vi "MM6.PG_Stop.vi"(0 "i ref in":refnum<vi>, 5 "error in (no error)":errorcluster) -> (14 "i ref out":refnum<vi>, 19 "error out":errorcluster)   [LabVIEW 2014, in "MM6.lvlib"]
doc: "Stops the hardware used for timing."
uses:
  MM6.lvlib
  CSCore/CSSystem/CoreLib/CoreLib.int 2 byte array.vi
  CSCore/BaseProcess/BaseProcess.lvlib
  CSCore/CSSystem/CoreLib/CoreLib.lvlib
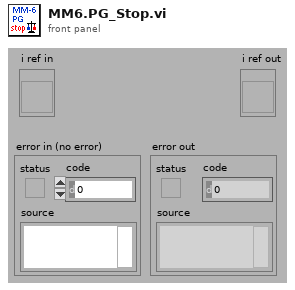
[diagram p1: front panel]
types:
  T1 = typedef "PPG_ABC.lvlib/PPG_ABC.PG_dataType.ctl" = cluster{"PGDevice":string, "rawPatternData":cluster{"triggerCondition":i32, "timeTable":dbl[], "channelTable":string[]}[]}
  T2 = typedef "CoreDefs.rawDataType.ctl" = i8[]
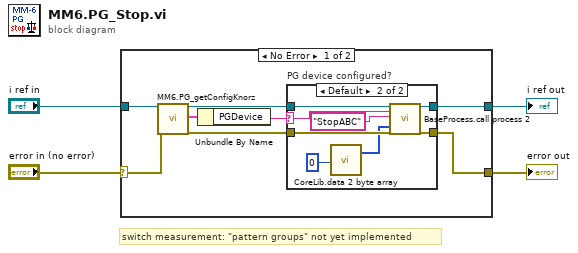
[diagram p0: block diagram]
diagram:
  # "switch measurement: \"pattern groups\" not yet implemented"
  n1 = case shown="No Error" "error in (no error)" {
    selector: "error in (no error)" -> [w11 w23]
    tunnel: "i ref in" -> [w12 w24]
    tunnel: [w7 w24] -> w3
    tunnel: [w6 w23] -> w2
    frame No Error {
      n2 = call "MM6.PG_getConfigKnorz.vi"("i ref in"=w12, "error in (no error)"=w11) -> ("i ref out"=w10:refnum<vi>, "PGData"=w8:T1, "error out"=w9:errorcluster)  [unwired: 15 in]
      n3 = Unbundle By Name(w8) -> ("PGDevice"=w5:string)
      n4 = case "PG device configured?" shown="Default" w5 {
        selector: w5 -> [_ w15]
        tunnel: w10 -> [w14 w22]
        tunnel: w9 -> [w13 w21]
        tunnel: [w14 w17] -> w7
        tunnel: [w13 w16] -> w6
        frame "" {
        }
        frame Default {
          n5 = call-poly "CoreLib.data 2 byte array.vi"("i32"=0) -> ("byteArray out"=w19:T2)  [unwired: 18 in]
          n6 = call "BaseProcess.call process 2.vi"("i ref in"=w22, "Object"=w15, "Selector"="StopABC", "Data"=w19, "error in (no error)"=w21) -> ("i ref out"=w17:refnum<vi>, "error out"=w16:errorcluster)  [unwired: 13 in]
        }
      }
    }
    frame Error {
    }
  }
  "error out" <- w2
  "i ref out" <- w3
